vi "力觉选择计算C.vi"(9 "力参数C":T1={"选择"=enum."Fx", "系数"=1.0, "上限"=4.3, "下限"=3.7, "Ymax"=50.0, "Ymin"=-50.0, "点数"=1000.0, "锁系数x"=1.0, "锁上限"=0.4, "锁下限"=0.6, "锁系数+"=1.0, "起点"=0.0, "终点"=0.0, "锁起点"=0.0, "锁终点"=0.0} {"锁终点" format="%.2f"; "锁起点" format="%.2f"; "终点" format="%.2f"; "起点" format="%.2f"; "锁系数+" format="%.3f"; "锁下限" format="%.2f"; "锁上限" format="%.2f"; "锁系数x" format="%.3f"; "下限" format="%.2f"; "上限" format="%.2f"; "系数" format="%.3f"}, 11 "力":sgl[](array[numeric]) format="%.2f") -> (1 "锁止":sgl, 3 "曲线":sgl)   [LabVIEW 2018]
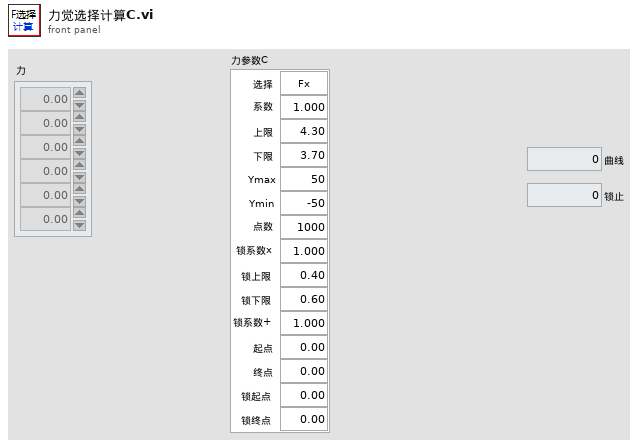
[diagram p1: front panel]
types:
  T1 = cluster{"选择":enum16{"Fx", "Fy", "Fz", "Mx", "My", "Mz"}, "系数":sgl, "上限":sgl, "下限":sgl, "Ymax":dbl, "Ymin":dbl, "点数":dbl, "锁系数x":sgl, "锁上限":sgl, "锁下限":sgl, "锁系数+":sgl, "起点":dbl, "终点":dbl, "锁起点":dbl, "锁终点":dbl}
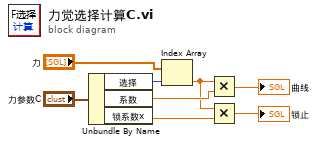
[diagram p0: block diagram]
diagram:
  n1 = Unbundle By Name("力参数C") -> ("选择"=w7:enum16{"Fx", "Fy", "Fz", "Mx", "My", "Mz"}, "系数"=w6:sgl, "锁系数x"=w4:sgl)
  n2 = Index Array(array="力", index=w7) -> (element=w5:sgl)
  n3 = Multiply(x=w5, y=w6) -> (x*y=→"曲线":sgl)
  n4 = Multiply(x=w5, y=w4) -> (x*y=→"锁止":sgl)
